vi "Read Value.vi"(8 "error in (no error)":errorcluster, 11 "Base in":refnum<class "KDemoBase.lvclass">) -> (0 "error out":errorcluster, 2 "Value":dbl, 3 "Base out":refnum<class "KDemoBase.lvclass">)   [LabVIEW 2015, in "KDemoBase.lvclass"]
uses:
  KDemoBase.lvclass
  KDemoBase.lvclass/KDemoBase.ctl
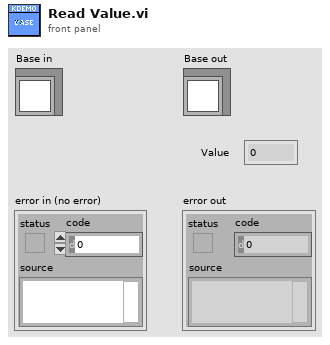
[diagram p1: front panel]
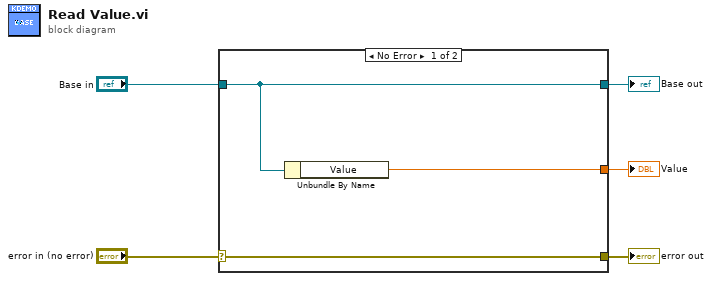
[diagram p0: block diagram]
diagram:
  n1 = case shown="No Error" "error in (no error)" {
    selector: "error in (no error)" -> [w8 w9]
    tunnel: [w8 w9] -> w4
    tunnel: [w7 w10] -> w2
    tunnel: "Base in" -> [w7 w10]
    tunnel: [w6 _] -> w1
    frame No Error {
      n2 = Unbundle By Name(w7) -> ("Value"=w6:dbl)
    }
    frame Error {
    }
  }
  "error out" <- w4
  "Base out" <- w2
  "Value" <- w1
